vi "VI Tree.vi"   [LabVIEW 2021, in "BK Precision 5491B.lvlib"]
doc: "This is the instrument driver for the BK Precision 5491B and 2831E. The VI Tree displays all the user-callable VIs of the instrument driver in an organized table."
uses:
  <instrlib>/BK Precision 5491B/BK Precision 5491B.lvlib
panel:
  # "(c) 2016 B&K Precision Corporation.  ALL RIGHTS RESERVED."
  # "SEE DIAGRAM\nFOR VI TREE."
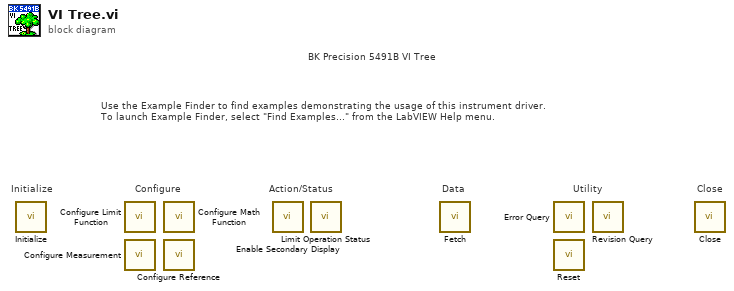
[diagram p0: block diagram]
diagram:
  # "BK Precision 5491B VI Tree"
  # "Action/Status"
  # "Use the Example Finder to find examples demonstrating the usage of this instrument driver.\nTo launch Example Finder, select \"Find Examples...\" from the LabVIEW Help menu."
  # "Configure"
  # "Utility"
  # "Data"
  # "Close"
  # "Initialize"
  n1 = call <instrlib>:"Initialize.vi"() -> ()  [unwired: 10 in, 2 out]
  n2 = call <instrlib>:"Configure Limit Function.vi"() -> ()  [unwired: 10 in, 2 out]
  n3 = call <instrlib>:"Configure Measurement.vi"() -> ()  [unwired: 10 in, 2 out]
  n4 = call <instrlib>:"Configure Math Function.vi"() -> ()  [unwired: 10 in, 2 out]
  n5 = call <instrlib>:"Configure Reference.vi"() -> ()  [unwired: 10 in, 2 out]
  n6 = call <instrlib>:"Enable Secondary Display.vi"() -> ()  [unwired: 10 in, 2 out]
  n7 = call <instrlib>:"Limit Operation Status.vi"() -> ()  [unwired: 9 in, 3 out]
  n8 = call <instrlib>:"Fetch.vi"() -> ()  [unwired: 8 in, 4 out]
  n9 = call <instrlib>:"Error Query.vi"() -> ()  [unwired: 9 in, 3 out]
  n10 = call <instrlib>:"Reset.vi"() -> ()  [unwired: 10 in, 2 out]
  n11 = call <instrlib>:"Revision Query.vi"() -> ()  [unwired: 8 in, 4 out]
  n12 = call <instrlib>:"Close.vi"() -> ()  [unwired: 11 in, 1 out]
